vi "MeasInductance.vi"() -> ()   [LabVIEW 2017]
uses:
  <vilib>/Analysis/6fits.llb/Curve Fitting Criteria.ctl
  <vilib>/Analysis/NI_AALPro.lvlib
  Keysight N8731A conversion/Keysight N8900 Series.lvlib
panel:
  out "Averaged Inductance":dbl
  in  "Measurements":i32=1
  in  "filename":string caption="Discard data if empty"
  out "Resistance (latest)":dbl
  out "Inductance (latest)":dbl
  out "V(I)":T1(graph)
  out "Time Data":dbl[](array[numeric])
  out "Voltage Data":dbl[](array[numeric])
  out "Current Data":dbl[](array[numeric])
  out "I(t)":T1(graph)
  in  "stop":bool
  out "start time":dbl format="%_19f"
  in  "Measurement time [s]":dbl=240.0
  in  "OV Value (10V)":dbl=10.0
  in  "VISA resource name":refnum<visa-resource-name>
  in  "Keithley (1)/PSU (0)":bool=TRUE caption="Voltage Source"
  in  "Voltage limit [V]":dbl
  in  "Current limit [A]":dbl
  in  "Time between measurements [ms]":dbl
  # "Program will set Voltage and Current to specified limits, then make\nmeasurements at specified intervals until the measurement is either\nmanually stopped or measurement time runs out. Once the\nmeasurement is over, Resistance and inductance are calculated, and\nthe coil is run down in two steps."
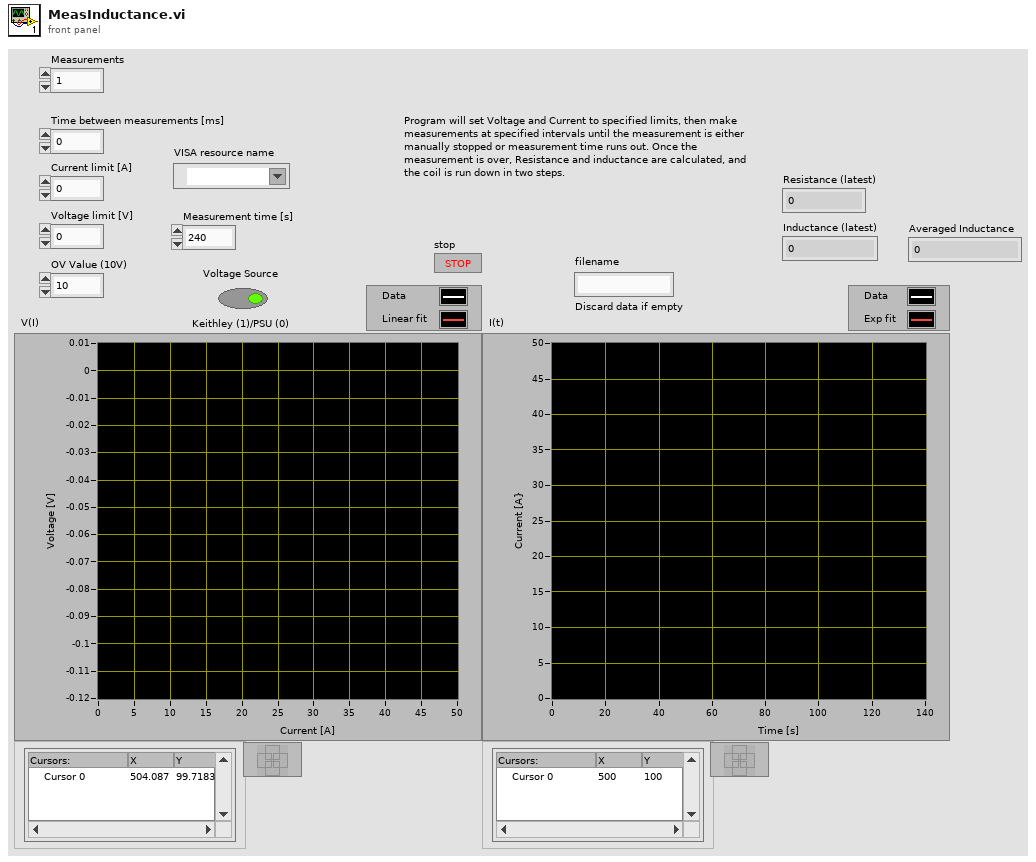
[diagram p1: front panel]
types:
  T1 = cluster{"Current Data":dbl[], "Best Linear Fit":dbl[]}[]
  T2 = cluster{"amp min":dbl, "amp max":dbl, "damping min":dbl, "damping max":dbl, "offset min":dbl, "offset max":dbl}
  T3 = typedef "NI_AALPro.lvlib/Curve Fitting Criteria.ctl" = u16
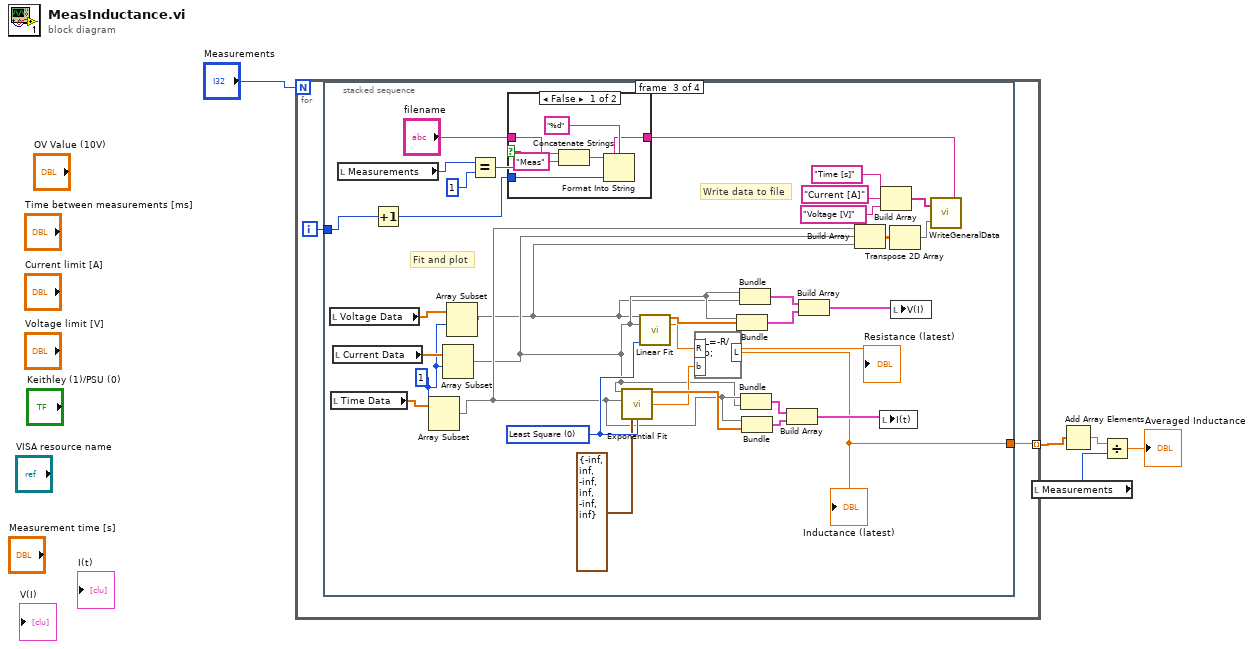
[diagram p0: block diagram]
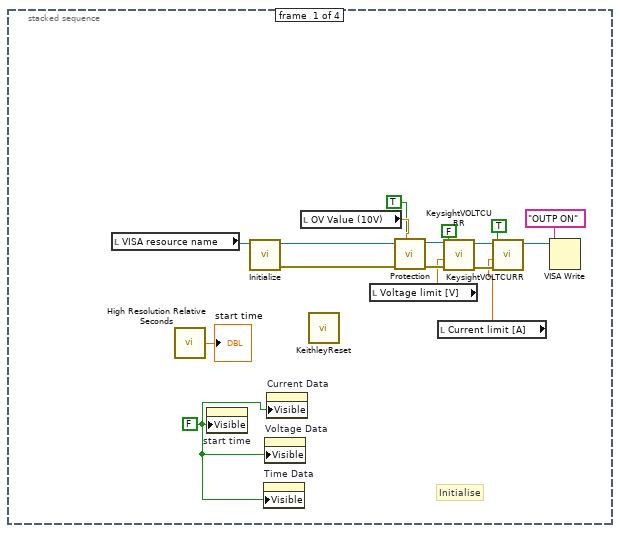
[diagram p2: hidden frame]
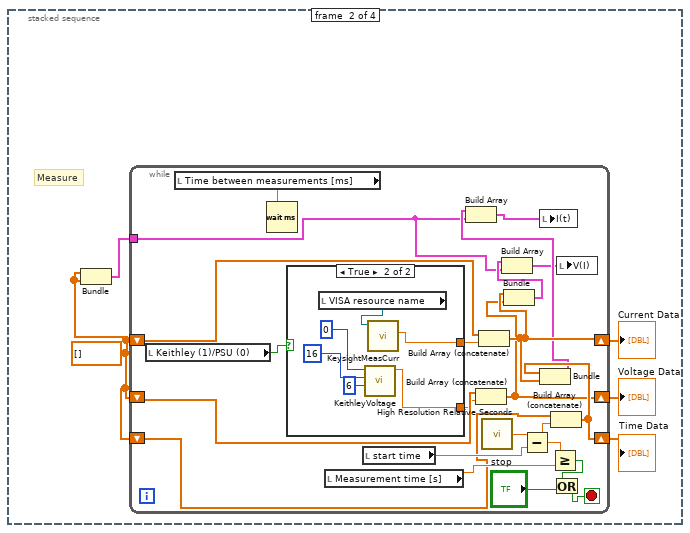
[diagram p3: hidden frame]
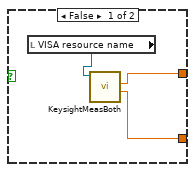
[diagram p4: hidden frame]
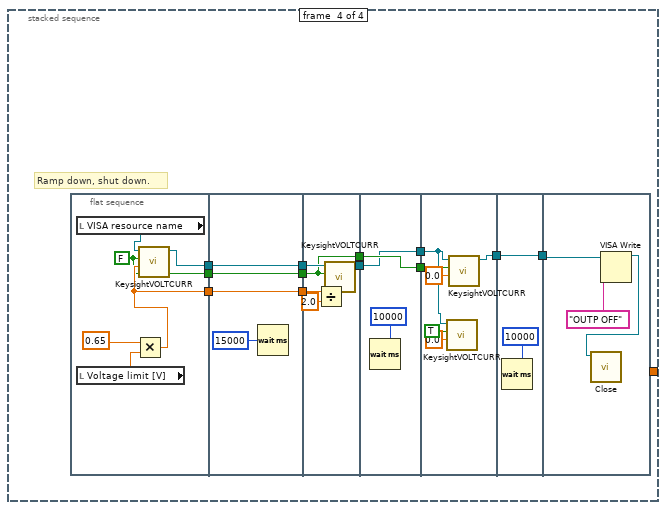
[diagram p6: hidden frame]
diagram:
  n1 = for {
    N: "Measurements" -> [_]
    tunnel: [w7] -> w3 mode=indexing
    i -> [w6]
    n2 = stacked-sequence {
      tunnel: [_ _ w68 _] -> w7
      tunnel: w6 -> [_ _ w62 _]
      frame #0 {
        w10 = FALSE ("Visible")
        # "Initialise"
        n3 = local read "VISA resource name"() -> (w22:refnum<visa-resource-name>)
        n4 = call <vilib>:"High Resolution Relative Seconds.vi"() -> ("relative seconds"=→"start time":dbl)
        n5 = property on="start time" class="DigNum (strict)"("Visible"=w10) -> ()  [unwired: 2 in, 2 out]
        n6 = call "Initialize.vi"("VISA resource name"=w22) -> ("error out"=w24:errorcluster, "VISA resource name out"=w23:refnum<visa-resource-name>)  [unwired: 9 in]
        n7 = property on="Time Data" class="Arr (strict)"("Visible"=w10) -> ()  [unwired: 2 in, 2 out]
        n8 = property on="Voltage Data" class="Arr (strict)"("Visible"=w10) -> ()  [unwired: 2 in, 2 out]
        n9 = property on="Current Data" class="Arr (strict)"("Visible"=w10) -> ()  [unwired: 2 in, 2 out]
        n10 = local read "OV Value (10V)"() -> (w21:dbl)
        n11 = call "KeithleyReset.vi"() -> ()  [unwired: 11 in, 1 out]
        n12 = local read "Voltage limit [V]"() -> (w12:dbl)
        n13 = call "Protection.vi"("OV protection"=TRUE, "error in (no error)"=w24, "OV Value (10V)"=w21, "VISA resource name"=w23) -> ("error out"=w18:errorcluster, "VISA resource name out"=w19:refnum<visa-resource-name>)  [unwired: 6 in]
        n14 = local read "Current limit [A]"() -> (w13:dbl)
        n15 = call "KeysightVOLTCURR.vi"("error in (no error)"=w18, "CURR/VOLT (A/V)"=w12, "CURR (1)/VOLT (0)"=FALSE, "VISA resource name"=w19) -> ("error out"=w15:errorcluster, "VISA resource name out"=w16:refnum<visa-resource-name>)  [unwired: 6 in]
        n16 = call "KeysightVOLTCURR.vi"("error in (no error)"=w15, "CURR/VOLT (A/V)"=w13, "CURR (1)/VOLT (0)"=TRUE, "VISA resource name"=w16) -> ("VISA resource name out"=w9:refnum<visa-resource-name>)  [unwired: 6 in, 1 out]
        n17 = VISA Write(VISA resource name=w9, write buffer="OUTP ON") -> ()  [unwired: 1 in, 3 out]
      }
      frame #1 {
        w26 = dbl[] []
        # "Measure"
        n18 = Bundle(w26, w26) -> (w25:cluster{dbl[], dbl[]})  [unwired: 1 in]
        n19 = while {
          shift-right: [w36] -> w29
          shift-left: w26 -> [w48]
          shift-right: [w35] -> w28
          shift-left: w26 -> [w49]
          shift-right: [w37] -> w27
          shift-left: w26 -> [w38]
          tunnel: w25 -> [w32]
          stop <- w40 stop-if-true
          n20 = local read "Keithley (1)/PSU (0)"() -> (w50:bool)
          n21 = local read "Time between measurements [ms]"() -> (w51:dbl)
          n22 = Wait (ms)(milliseconds to wait=w51) -> ()  [unwired: 1 out]
          n23 = case shown="True" w50 {
            tunnel: [w53 w60] -> w47
            tunnel: [w52 w59] -> w46
            frame False {
              n24 = local read "VISA resource name"() -> (w54:refnum<visa-resource-name>)
              n25 = call "KeysightMeasBoth.vi"("VISA resource name"=w54) -> ("VOLT"=w52:dbl, "CURR"=w53:dbl)  [unwired: 7 in, 2 out]
            }
            frame True {
              n26 = local read "VISA resource name"() -> (w58:refnum<visa-resource-name>)
              n27 = call "KeithleyVoltage.vi"("channel (6)"=6, "address (16)"=i16 16, "bus"=0) -> ("Voltage"=w59:dbl)  [unwired: 7 in, 1 out]
              n28 = call "KeysightMeasCurr.vi"("VISA resource name"=w58) -> ("CURR"=w60:dbl)  [unwired: 8 in, 2 out]
            }
          }
          n29 = local read "Measurement time [s]"() -> (w43:dbl)
          n30 = local read "start time"() -> (w44:dbl)
          n31 = Build Array (concatenate)(w49, w46) -> (w35:dbl[])
          n32 = Build Array (concatenate)(w48, w47) -> (w36:dbl[])
          n33 = call <vilib>:"High Resolution Relative Seconds.vi"() -> ("relative seconds"=w45:dbl)
          n34 = Bundle(w36, w35) -> (w33:cluster{dbl[], dbl[]})  [unwired: 1 in]
          n35 = Build Array(w33, w32) -> (w30:cluster{dbl[], dbl[]}[])
          n36 = Subtract(x=w45, y=w44) -> (x-y=w39:dbl)
          n37 = Greater Or Equal?(x=w39, y=w43) -> (x >= y?=w42:bool)
          n38 = Build Array (concatenate)(w38, w39) -> (w37:dbl[])
          n39 = Bundle(w37, w36) -> (w34:cluster{dbl[], dbl[]})  [unwired: 1 in]
          n40 = Build Array(w34, w32) -> (w31:cluster{dbl[], dbl[]}[])
          n41 = local write "I(t)"(w31) -> ()
          n42 = Or(x=w42, y="stop") -> (x .or. y?=w40:bool)
          n43 = local write "V(I)"(w30) -> ()
        }
        "Current Data" <- w29
        "Voltage Data" <- w28
        "Time Data" <- w27
      }
      frame #2 {
        w69 = 1 ("index")
        w93 = T3 0 items=["Least Square", "Least Absolute Residual", "Bisquare"] ("method")
        # "Write data to file"
        # "Fit and plot"
        n44 = local read "Voltage Data"() -> (w71:dbl[])
        n45 = local read "Time Data"() -> (w75:dbl[])
        n46 = local read "Current Data"() -> (w73:dbl[])
        n47 = local read "Measurements"() -> (w64:i32)
        n48 = Increment(x=w62) -> (x+1=w61:i32)
        n49 = Array Subset(array=w75, index=w69) -> (w74:dbl[])  [unwired: 1 in]
        n50 = Array Subset(array=w73, index=w69) -> (w72:dbl[])  [unwired: 1 in]
        n51 = Array Subset(array=w71, index=w69) -> (w70:dbl[])  [unwired: 1 in]
        n52 = Equal?(x=w64, y=1) -> (x = y?=w66:bool)
        n53 = case shown="False" w66 {
          tunnel: "filename" -> [w96 w100]
          tunnel: [w97 w100] -> w65
          tunnel: w61 -> [w98 _]
          frame False {
            n54 = Concatenate Strings(w96, "Meas" ("string")) -> (w94:string)
            n55 = Format Into String(format string="%d", initial string=w94, w98) -> (resulting string=w97:string)  [unwired: 1 in, 1 out]
          }
          frame True {
          }
        }
        n56 = call <vilib>:"Exponential Fit.vi"("Y"=w72, "X"=w74, "method"=w93, "parameter bounds"=T2 {"amp min"=-inf, "amp max"=inf, "damping min"=-inf, "damping max"=inf, "offset min"=-inf, "offset max"=inf}) -> ("Best Exponential Fit"=w87:dbl[], "damping"=w82:dbl)  [unwired: 6 in, 4 out]
        n57 = call <vilib>:"Linear Fit.vi"("Y"=w70, "X"=w72, "method"=w93) -> ("Best Linear Fit"=w92:dbl[], "slope"=w83:dbl)  [unwired: 8 in, 3 out]
        "Resistance (latest)" <- w83
        n58 = formula code="L=-R/b;"("b"=w82, "R"=w83) -> ("L"=w68:dbl)
        "Inductance (latest)" <- w68
        n59 = Bundle(w72, "Best Linear Fit"=w92) -> (w89:cluster{dbl[], "Best Linear Fit":dbl[]})  [unwired: 1 in]
        n60 = Bundle(w72, w70) -> (w88:cluster{dbl[], dbl[]})  [unwired: 1 in]
        n61 = Bundle(w74, w72) -> (w91:cluster{dbl[], dbl[]})  [unwired: 1 in]
        n62 = Bundle(w74, "Best Exponential Fit"=w87) -> (w90:cluster{dbl[], "Best Exponential Fit":dbl[]})  [unwired: 1 in]
        n63 = Build Array(w91, w90) -> (w85:cluster{dbl[], "Best Exponential Fit":dbl[]}[])
        n64 = Build Array(w88, w89) -> (w86:cluster{dbl[], "Best Linear Fit":dbl[]}[])
        n65 = Build Array(w74, w72, w70) -> (w77:dbl[][])
        n66 = local write "I(t)"(w85) -> ()
        n67 = Build Array("Time [s]", "Current [A]", "Voltage [V]") -> (w78:string[])
        n68 = Transpose 2D Array(2D array=w77) -> (transposed array=w76:dbl[][])
        n69 = local write "V(I)"(w86) -> ()
        n70 = call "WriteGeneralData.vi"("filename (discard if empty)"=w65, "Array"=w76, "Column name array"=w78) -> ()
      }
      frame #3 {
        # "Ramp down, shut down."
        n71 = flat-sequence {
          tunnel: [w115] -> w111
          tunnel: [w114] -> w109
          tunnel: [w113] -> w107
          tunnel: [w121] -> w112
          tunnel: w111 -> [w121]
          tunnel: [w120] -> w110
          tunnel: w109 -> [w120]
          tunnel: [w119] -> w108
          tunnel: w107 -> [w119]
          tunnel: w112 -> [w128]
          tunnel: w110 -> [w126]
          tunnel: w108 -> [w124]
          tunnel: [w124] -> w105
          tunnel: [w123] -> w103
          tunnel: [w130] -> w106
          tunnel: w105 -> [w130]
          tunnel: [w129] -> w104
          tunnel: w103 -> [w129]
          tunnel: w106 -> [w137]
          tunnel: w104 -> [w134]
          tunnel: [w132] -> w102
          tunnel: w102 -> [w139]
          tunnel: [w139] -> w101
          tunnel: w101 -> [w142]
          frame #0 {
            w113 = FALSE ("CURR (1)/VOLT (0)")
            n72 = local read "VISA resource name"() -> (w118:refnum<visa-resource-name>)
            n73 = local read "Voltage limit [V]"() -> (w117:dbl)
            n74 = Multiply(x=0.65, y=w117) -> (x*y=w114:dbl)
            n75 = call "KeysightVOLTCURR.vi"("CURR/VOLT (A/V)"=w114, "CURR (1)/VOLT (0)"=w113, "VISA resource name"=w118) -> ("VISA resource name out"=w115:refnum<visa-resource-name>)  [unwired: 7 in, 1 out]
          }
          frame #1 {
            n76 = Wait (ms)(milliseconds to wait=u32 15000) -> ()  [unwired: 1 out]
          }
          frame #2 {
            n77 = Divide(x=w126, y=2.0) -> (x/y=w125:dbl)
            n78 = call "KeysightVOLTCURR.vi"("CURR/VOLT (A/V)"=w125, "CURR (1)/VOLT (0)"=w124, "VISA resource name"=w128) -> ("VISA resource name out"=w123:refnum<visa-resource-name>)  [unwired: 7 in, 1 out]
          }
          frame #3 {
            n79 = Wait (ms)(milliseconds to wait=u32 10000) -> ()  [unwired: 1 out]
          }
          frame #4 {
            n80 = call "KeysightVOLTCURR.vi"("CURR/VOLT (A/V)"=0.0, "CURR (1)/VOLT (0)"=TRUE, "VISA resource name"=w134) -> ()  [unwired: 7 in, 2 out]
            n81 = call "KeysightVOLTCURR.vi"("CURR/VOLT (A/V)"=0.0, "CURR (1)/VOLT (0)"=w137, "VISA resource name"=w134) -> ("VISA resource name out"=w132:refnum<visa-resource-name>)  [unwired: 7 in, 1 out]
          }
          frame #5 {
            n82 = Wait (ms)(milliseconds to wait=u32 10000) -> ()  [unwired: 1 out]
          }
          frame #6 {
            n83 = VISA Write(VISA resource name=w142, write buffer="OUTP OFF") -> (VISA resource name out=w140:refnum<visa-resource-name>)  [unwired: 1 in, 2 out]
            n84 = call "Close.vi"("VISA resource name"=w140) -> ()  [unwired: 10 in, 1 out]
          }
        }
      }
    }
  }
  n85 = local read "Measurements"() -> (w4:i32)
  n86 = Add Array Elements(numeric array=w3) -> (sum=w2:dbl)
  n87 = Divide(x=w2, y=w4) -> (x/y=→"Averaged Inductance":dbl)
